vi "GDSLvIcon_GenerateIconText.vi"(1 "Text":T2, 2 "TextPixelHeight(5-30)":i32=7, 3 "Foreground color":u32(colorbox), 4 "Background color":u32(colorbox)=16777215, 5 "error in (no error)":errorcluster, 6 "Offset":cluster{"X":i32, "Y":i32}, 7 "Text Pixel width(32-FrameThicknes*2))":i32=30) -> (14 "X-Limited":bool, 15 "Y-Limited":bool, 17 "TextOut":u8[][](array[numeric]), 18 "TextBounds":T1, 19 "error out":errorcluster)   [LabVIEW 2020]
doc: "Applies a text in the template picture."
uses:
  GDSLvIcon_TextDataType.ctl
  GDSLvIcon_WordCompressionType.ctl
  GDSLvIcon_TextAlignment.ctl
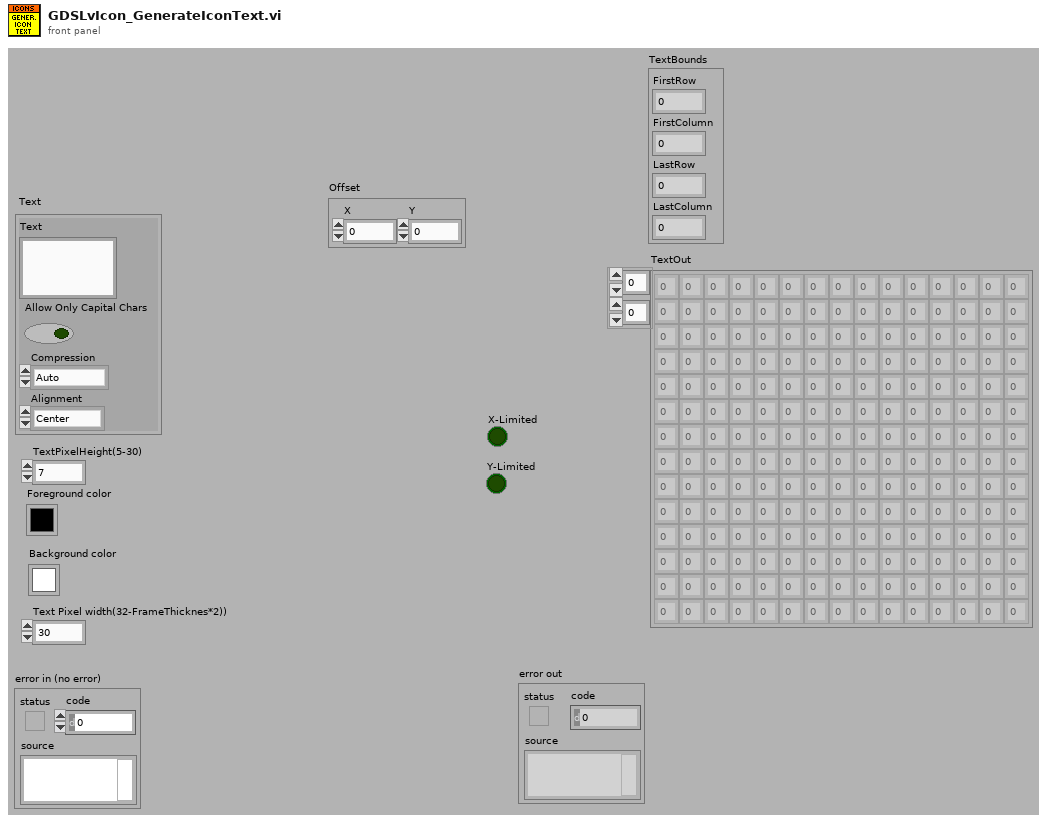
[diagram p1: front panel]
types:
  T1 = cluster{"FirstRow":i32, "FirstColumn":i32, "LastRow":i32, "LastColumn":i32}
  T2 = typedef "GDSLvIcon_TextDataType.ctl" = cluster{"Text":string, "Allow Only Capital Chars":bool, "Compression":T3, "Alignment":T4}
  T3 = typedef "GDSLvIcon_WordCompressionType.ctl" = enum16{"Auto", "On", "Off"}
  T4 = typedef "GDSLvIcon_TextAlignment.ctl" = enum16{"Center", "Left", "Right"}
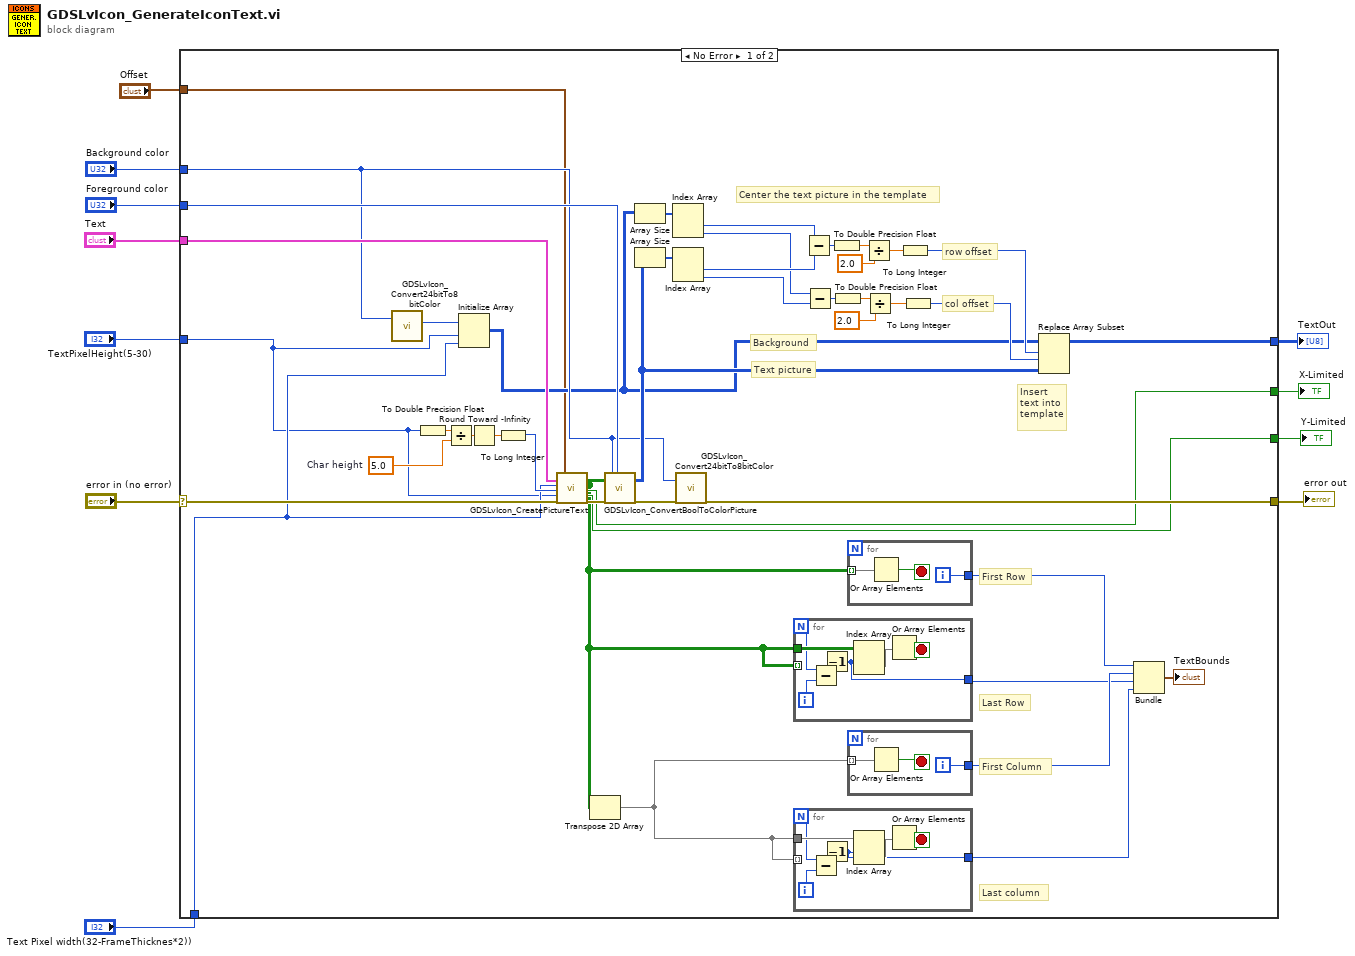
[diagram p0: block diagram]
diagram:
  n1 = case shown="No Error" "error in (no error)" {
    selector: "error in (no error)" -> [w31 w76]
    tunnel: [w33 w76] -> w10
    tunnel: "Foreground color" -> [w34 _]
    tunnel: "Background color" -> [w26 _]
    tunnel: "Text" -> [w55 _]
    tunnel: "TextPixelHeight(5-30)" -> [w22 _]
    tunnel: [w23 _] -> w5
    tunnel: "Text Pixel width(32-FrameThicknes*2))" -> [w25 _]
    tunnel: "Offset" -> [w21 _]
    tunnel: [w20 _] -> w2
    tunnel: [w19 _] -> w1
    frame No Error {
      w54 = 5.0  # Char height
      # "Last column"
      # "First Column"
      # "Last Row"
      # "First Row"
      # "Insert\ntext into\ntemplate"
      # "col offset"
      # "row offset"
      # "Center the text picture in the template"
      # "Text picture"
      # "Background"
      n2 = call "GDSLvIcon_Convert24bitTo8bitColor.vi"("Color 24bit In"=w26) -> ("Color out(256)"=w32:u8)  [unwired: 15 in, 3 out]
      n3 = To Double Precision Float(number=w22) -> (double precision float=w53:dbl)
      n4 = Divide(x=w53, y=w54) -> (x/y=w52:dbl)
      n5 = Initialize Array(w32, w22, w25) -> (w24:u8[][])
      n6 = Round Toward -Infinity(1:w52) -> (0:w51:dbl)
      n7 = To Long Integer(number=w51) -> (32bit integer=w50:i32)
      n8 = call "GDSLvIcon_CreatePictureText.vi"("Text"=w55, "Pixel width"=w25, "Max nr of rows"=w50, "Pixel height"=w22, "error in (no error)"=w31, "Offset"=w21) -> ("CharPicture"=w15:bool[][], "X-Limited"=w20:bool, "Y-Limited"=w19:bool, "error out"=w36:errorcluster)  [unwired: 10 in]
      n9 = Transpose 2D Array(2D array=w15) -> (transposed array=w14:bool[][])
      n10 = call "GDSLvIcon_ConvertBoolToColorPicture.vi"("CharPicture"=w15, "error in (no error)"=w36, "Background color"=w26, "Foreground color"=w34) -> ("CharPicture out"=w27:u8[][], "error out"=w35:errorcluster)  [unwired: 14 in]
      n11 = Array Size(array=w24) -> (size(s)=w30:i32[])
      n12 = Array Size(array=w27) -> (size(s)=w49:i32[])
      n13 = Index Array(array=w30) -> (element #1=w29:i32, element #2=w28:i32)  [unwired: 2 in]
      n14 = Index Array(array=w49) -> (element #1=w48:i32, element #2=w41:i32)  [unwired: 2 in]
      n15 = call "GDSLvIcon_Convert24bitTo8bitColor.vi"("Color 24bit In"=w26, "error in (no error)"=w35) -> ("error out"=w33:errorcluster)  [unwired: 14 in, 3 out]
      n16 = for {
        N -> [w70]
        tunnel: w15 -> [w71]
        tunnel: [w66] -> w16
        tunnel: w15 -> [_] mode=indexing
        i -> [w69]
        stop <- w72 stop-if-true
        n17 = Subtract(x=w70, y=w69) -> (x-y=w68:i32)
        n18 = Decrement(x=w68) -> (x-1=w66:i32)
        n19 = Index Array(array=w71, index (row)=w66) -> (element=w67:bool[])  [unwired: 1 in]
        n20 = Or Array Elements(Boolean array=w67) -> (logical OR=w72:bool)
      }
      n21 = for {
        N -> [w60]
        tunnel: w14 -> [w61]
        tunnel: w14 -> [_] mode=indexing
        tunnel: [w56] -> w13
        i -> [w59]
        stop <- w62 stop-if-true
        n22 = Subtract(x=w60, y=w59) -> (x-y=w58:i32)
        n23 = Decrement(x=w58) -> (x-1=w56:i32)
        n24 = Index Array(array=w61, index (row)=w56) -> (element=w57:bool[])  [unwired: 1 in]
        n25 = Or Array Elements(Boolean array=w57) -> (logical OR=w62:bool)
      }
      n26 = Subtract(x=w29, y=w48) -> (x-y=w47:i32)
      n27 = Subtract(x=w28, y=w41) -> (x-y=w42:i32)
      n28 = To Double Precision Float(number=w47) -> (double precision float=w45:dbl)
      n29 = To Double Precision Float(number=w42) -> (double precision float=w44:dbl)
      n30 = for {
        tunnel: w15 -> [w75] mode=indexing
        tunnel: [w73] -> w18
        i -> [w73]
        stop <- w74 stop-if-true
        n31 = Or Array Elements(Boolean array=w75) -> (logical OR=w74:bool)
      }
      n32 = for {
        tunnel: w14 -> [w65] mode=indexing
        tunnel: [w63] -> w17
        i -> [w63]
        stop <- w64 stop-if-true
        n33 = Or Array Elements(Boolean array=w65) -> (logical OR=w64:bool)
      }
      n34 = Divide(x=w45, y=2.0) -> (x/y=w40:dbl)
      n35 = Divide(x=w44, y=2.0) -> (x/y=w39:dbl)
      n36 = To Long Integer(number=w40) -> (32bit integer=w38:i32)
      n37 = To Long Integer(number=w39) -> (32bit integer=w37:i32)
      n38 = Replace Array Subset(array=w24, new element=w27, index (row)=w38, index (col)=w37) -> (w23:u8[][])
      n39 = Bundle(w18, w17, w16, w13) -> (→"TextBounds":cluster{i32, i32, i32, i32})  [unwired: 1 in]
    }
    frame Error {
    }
  }
  "error out" <- w10
  "TextOut" <- w5
  "Y-Limited" <- w1
  "X-Limited" <- w2
